vi "Main.vi"(11 "Module Admin":refnum<class "Delacor_lib_QMH_Module Admin.lvclass">) -> ()   [LabVIEW 2019, in "Settings Editor.lvlib"]
doc: "This template is based off of the Queued Message Handler design pattern and the Queued Message Handler project template that ships with LabVIEW.\n\nThe main difference is that the queue is private to this module and communication between modules is performed via Broadcast and Request events.\n\nRequest events are wrapped in public API methods and are handled in the Event Handling Loop (EHL) of this VI. Any module can register for Broadcast events sent by this module. The EHL generates messages based on user interface actions.\n\nThe Message Handling Loop (MHL) processes messages generated by the EHL, or by other messages. The messages are string values, so new messages can be added easily to the Message Cases case structure in the MHL. Each message cluster can also provide an optional value for Message Data, which is a variant that can be converted to whatever message-specific data is required.\n_____\nBased on Delacor QMH Project Template 4.0.0.47.\n_____\nBased on DQMH Project Template 6.1.0.94."
uses:
  Settings Editor.lvlib
  <vilib>/Delacor/Delacor QMH/Libraries/Module Admin_class/Delacor_lib_QMH_Module Admin.lvclass
  Module Data--cluster.ctl
  Settings--cluster.ctl
  Stop Argument--cluster.ctl
  <vilib>/Delacor/Delacor QMH/Libraries/Message Queue_class/Delacor_lib_QMH_Message Queue.lvclass/Delacor_lib_QMH_Message Queue.ctl
  <vilib>/Delacor/Delacor QMH/Libraries/Module Admin_class/Delacor_lib_QMH_Module Admin.lvclass/Delacor_lib_QMH_Module Admin.ctl
  <vilib>/Utility/miscctls.llb/LVPointTypeDef.ctl
  <vilib>/Delacor/Delacor QMH/Libraries/Message Queue_class/Delacor_lib_QMH_Enqueue Message (Single).vi
  <vilib>/Delacor/Delacor QMH/Libraries/Module Admin_class/Delacor_lib_QMH_Get External Launch.vi
  <vilib>/Utility/error.llb/Error Cluster From Error Code.vi
  <vilib>/ErrorRing/Error Ring.xnode
  <vilib>/Delacor/Delacor QMH/Libraries/Message Queue_class/Delacor_lib_QMH_Message Queue.lvclass
panel:
  in  "Dir?":bool=TRUE
  in  "TDMS Directory":path
  in  "Cancel":bool
  in  "OK":bool
  in  "TDMS filepath":path
  out "error out":errorcluster
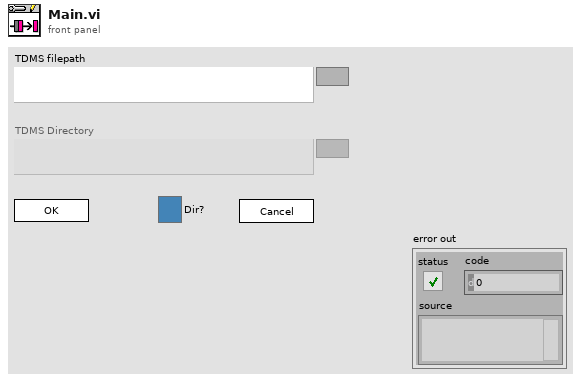
[diagram p1: front panel]
types:
  T1 = typedef "Settings Editor.lvlib/Request Events--cluster.ctl" = cluster{"Stop Module":refnum<user-event>, "Show Panel":refnum<user-event>, "Hide Panel":refnum<user-event>, "Get Module Execution Status":refnum<user-event>, "Show Diagram":refnum<user-event>}
  T2 = typedef "Settings Editor.lvlib/Module Data--cluster.ctl" = cluster{"Settings":T3}
  T3 = typedef "Settings Editor.lvlib/Settings--cluster.ctl" = cluster{"TDMS Filepath":path, "TDMS Directory":path}
  T4 = enum32{"invalid lock state", "Not Locked", "Locked (No Password)", "Password-protected"}
  T5 = typedef "Settings Editor.lvlib/Stop Argument--cluster.ctl" = cluster{"Origin":string, "Exit via Stop Module Req?":bool, "Wait for Module to stop?":bool}
  T6 = typedef "LVPointTypeDef.ctl" = cluster{"Horizontal":i16, "Vertical":i16}
  T7 = enum32{"Invalid", "Standard", "Closed", "Hidden", "Minimized", "Maximized"}
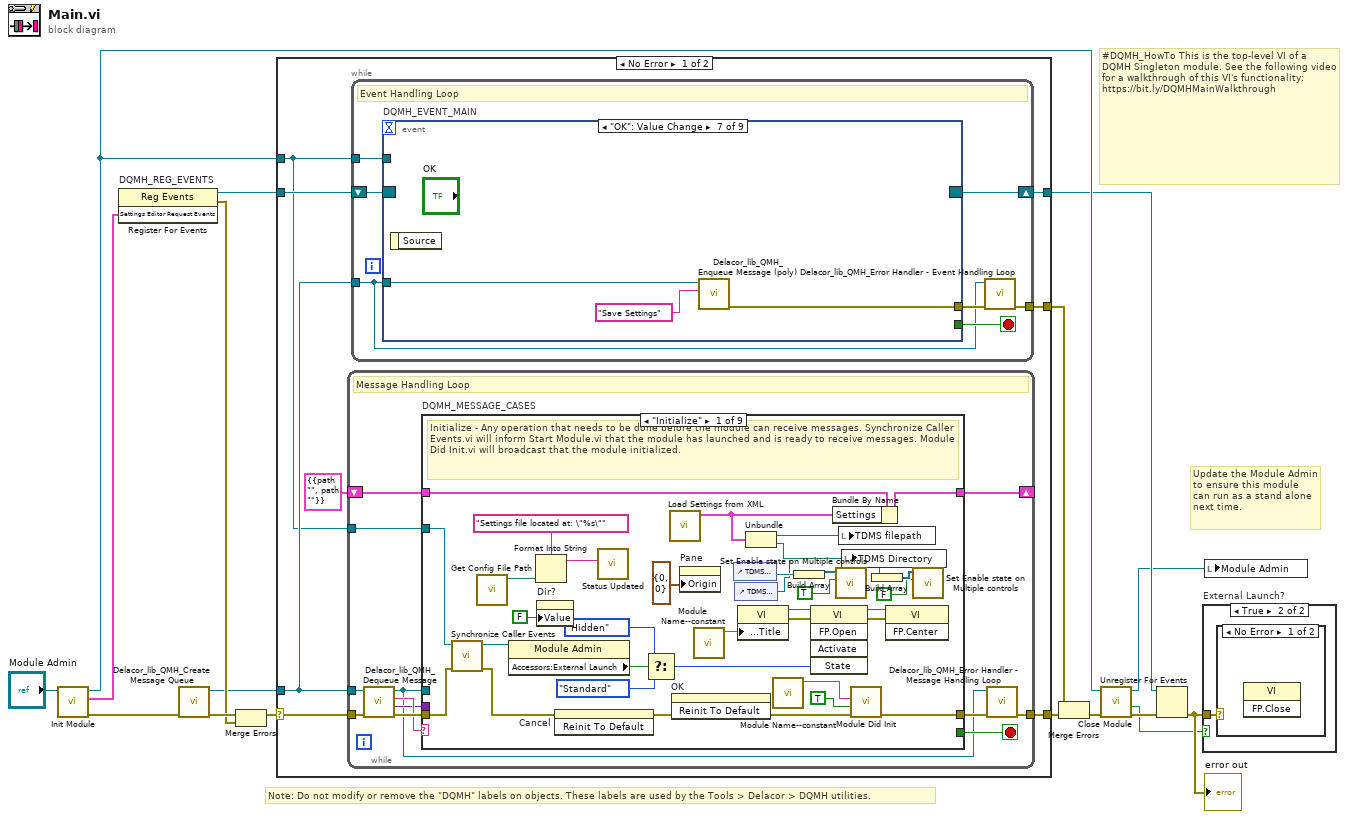
[diagram p0: block diagram]
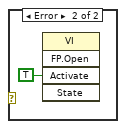
[diagram p3: hidden frame]
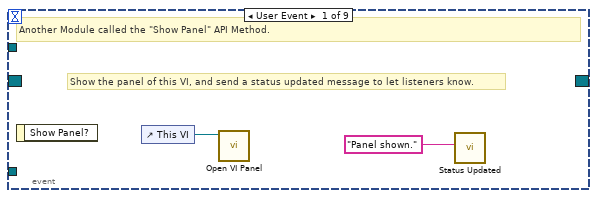
[diagram p4: hidden frame]
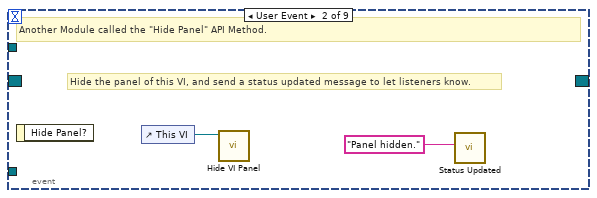
[diagram p5: hidden frame]
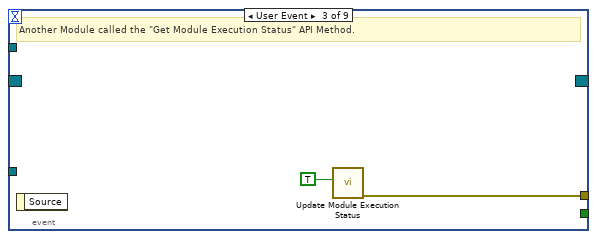
[diagram p6: hidden frame]
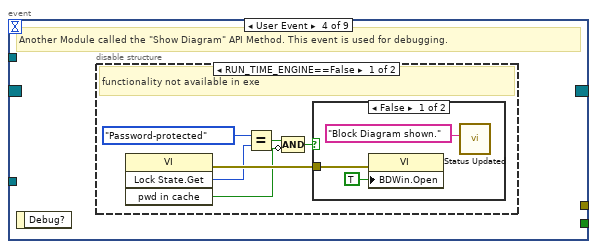
[diagram p7: hidden frame]
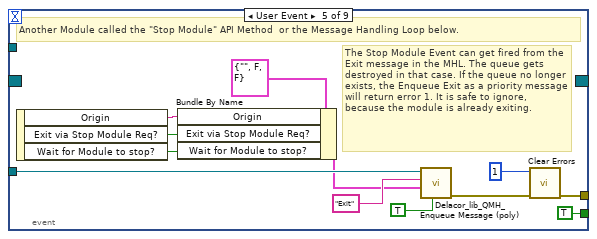
[diagram p10: hidden frame]
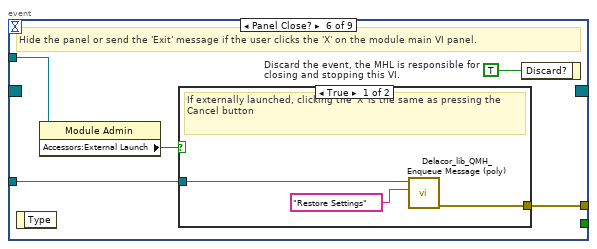
[diagram p11: hidden frame]
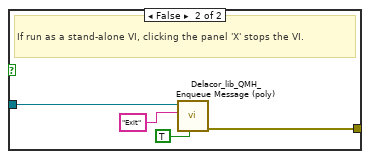
[diagram p12: hidden frame]
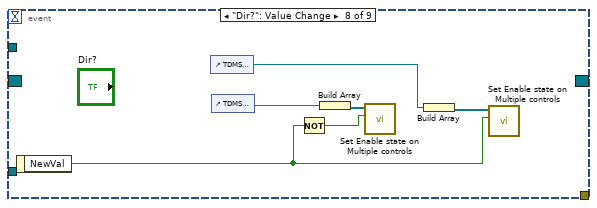
[diagram p13: hidden frame]
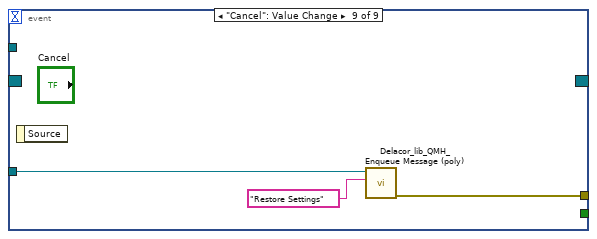
[diagram p14: hidden frame]
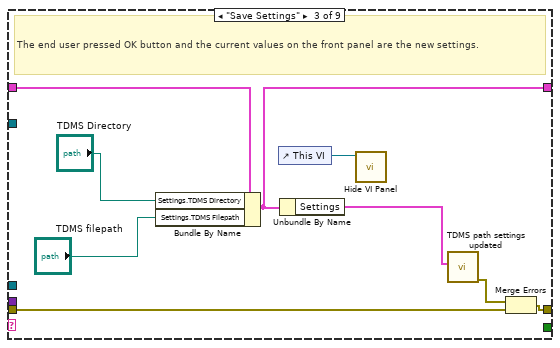
[diagram p16: hidden frame]
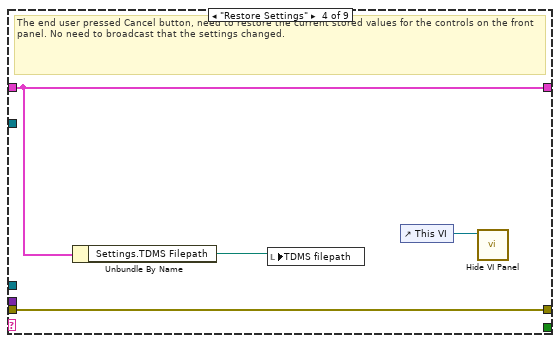
[diagram p17: hidden frame]
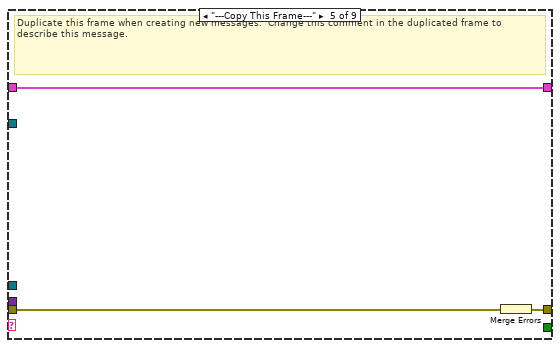
[diagram p18: hidden frame]
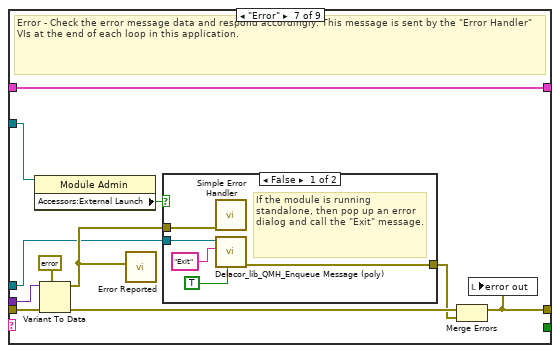
[diagram p20: hidden frame]
diagram:
  # "#DQMH_HowTo This is the top-level VI of a DQMH Singleton module. See the following video for a walkthrough of this VI's functionality: https://bit.ly/DQMHMainWalkthrough"
  # "Note: Do not modify or remove the \"DQMH\" labels on objects. These labels are used by the Tools > Delacor > DQMH utilities."
  # "Update the Module Admin to ensure this module can run as a stand alone next time."
  n1 = call "Init Module.vi"("Singleton Module Admin in"="Module Admin") -> ("error out"=w16:errorcluster, "Settings Editor Request Events"=w5:T1, "Singleton Module Admin out"=w8:refnum<class "Delacor_lib_QMH_Module Admin.lvclass">)  [unwired: 8 in]
  n2 = register-events "DQMH_REG_EVENTS"(w5) -> (reference out=w6:refnum<event-registration>, error out=w9:errorcluster)  [unwired: 2 in]
  n3 = call <vilib>:"Delacor_lib_QMH_Create Message Queue.vi"("error in"=w16) -> ("error out"=w11:errorcluster, "Message Queue"=w4:refnum<class "Delacor_lib_QMH_Message Queue.lvclass">)  [unwired: 9 in]
  n4 = Merge Errors(w11, w9) -> (w10:errorcluster)
  n5 = case shown="No Error" w10 {
    selector: w10 -> [w23 w194]
    tunnel: [w25 w193] -> w17
    tunnel: [w22 w200] -> w7
    tunnel: w6 -> [w20 w200]
    tunnel: w4 -> [w19 w195]
    tunnel: [w24 _] -> w14
    tunnel: w8 -> [w18 w196]
    frame No Error {
      n6 = while {
        tunnel: w19 -> [w86]
        shift-right: [w90] -> _
        shift-left: T2 {"Settings"={"TDMS Filepath"=path "", "TDMS Directory"=path ""}} ("Data Cluster") -> [w91]
        tunnel: w23 -> [w94]
        tunnel: [w92] -> w25
        tunnel: w18 -> [w84]
        stop <- w89 stop-if-true
        # "Message Handling Loop"
        n7 = call-dynamic "Delacor_lib_QMH_Dequeue Message.vi"("error in"=w94, "Message Queue in"=w86) -> ("error out"=w93:errorcluster, "Message Data"=w87:variant, "Message"=w88:string, "Message Queue out"=w85:refnum<class "Delacor_lib_QMH_Message Queue.lvclass">)  [unwired: 6 in]
        n8 = case "DQMH_MESSAGE_CASES" shown="\"Initialize\"" w88 {
          selector: w88 -> [_ _ _ _ _ _ _ _ w180]
          tunnel: w85 -> [_ _ _ _ _ _ w150 w172 _]
          tunnel: w93 -> [w126 w129 w133 w142 w145 w147 w157 w178 w182]
          tunnel: [w124 w129 w134 w142 w144 w147 w153 w175 w183] -> w95
          tunnel: w91 -> [w115 w128 w138 w141 w143 w146 w152 w171 w181]
          tunnel: [w114 w128 w136 w141 w143 w146 w152 w171 w181] -> w90
          tunnel: [_ _ _ _ _ _ _ w170 _] -> w89
          tunnel: w87 -> [_ _ _ _ _ _ w151 w169 _]
          tunnel: w84 -> [w116 _ _ _ _ _ w149 w164 _]
          frame "Initialize" {
            # "Initialize - Any operation that needs to be done before the module can receive messages. Synchronize Caller Events.vi will inform Start Module.vi that the module has launched and is ready to receive messages. Module Did Init.vi will broadcast that the module initialized."
            n9 = call "Synchronize Caller Events.vi"("error in (no error)"=w126, "Singleton Module Admin in"=w116) -> ("error out"=w125:errorcluster, "Singleton Module Admin out"=w111:refnum<class "Delacor_lib_QMH_Module Admin.lvclass">)  [unwired: 8 in]
            n10 = call "Get Config File Path.vi"() -> ("XML File Path"=w108:path)  [unwired: 10 in, 1 out]
            n11 = property class="Module Admin"(reference=w111) -> ("Accessors:External Launch"=w120:bool)  [unwired: 1 in, 2 out]
            n12 = Format Into String(format string="Settings file located at: \"%s\"", w108) -> (resulting string=w107:string)  [unwired: 2 in, 1 out]
            n13 = property on="Dir?" class="Bool (strict)"("Value"=FALSE ("Dir?")) -> ()  [unwired: 2 in, 2 out]
            n14 = invoke on="Cancel" class="Bool" method="Reinit To Default"() -> ()  [unwired: 3 in, 3 out]
            n15 = call "Status Updated.vi"("Status"=w107) -> ()  [unwired: 10 in, 1 out]
            n16 = Select(t=T7."Hidden" ("State"), s=w120, f=T7."Standard" ("State")) -> (s? t:f=w117:T7)
            n17 = call "Load Settings from XML.vi"() -> ("Settings out"=w105:T3)  [unwired: 10 in, 1 out]
            n18 = invoke on="OK" class="Bool" method="Reinit To Default"() -> ()  [unwired: 3 in, 3 out]
            n19 = property on="Pane" class="Pane"("Origin"=T6 {"Horizontal"=0, "Vertical"=0}) -> ()  [unwired: 2 in, 2 out]
            n20 = call "Module Name--constant.vi"() -> ("Module Name"=w123:string)  [unwired: 11 in]
            n21 = control-ref of="TDMS filepath"() -> (w102:refnum<vi>)
            n22 = control-ref of="TDMS Directory"() -> (w101:refnum<vi>)
            n23 = property class="VI"("Front Panel.Title"=w123) -> (reference out=w122:refnum<vi>, error out=w109:errorcluster)  [unwired: 2 in]
            n24 = Unbundle(w105) -> ("TDMS Filepath"=w104:path, "TDMS Directory"=w103:path)
            n25 = call "Module Name--constant.vi"() -> ("Module Name"=w112:string)  [unwired: 11 in]
            n26 = Build Array(w102) -> (w100:refnum<vi>[])
            n27 = invoke class="VI" method="FP.Open"(reference=w122, error in=w109, "State"=w117) -> (reference out=w121:refnum<vi>, error out=w127:errorcluster)  [unwired: 2 in, 3 out]
            n28 = Bundle By Name(cluster=w115, "Settings"=w105) -> (w114:T2)
            n29 = call "Set Enable state on Multiple controls.vi"("Enable?"=TRUE, "Controls"=w100) -> ()  [unwired: 10 in]
            n30 = local write "TDMS filepath"(w104) -> ()
            n31 = local write "TDMS Directory"(w103) -> ()
            n32 = call "Module Did Init.vi"("error in (no error)"=w125, "Initialized?"=TRUE, "Origin"=w112) -> ("error out"=w124:errorcluster)  [unwired: 8 in]
            n33 = Build Array(w101) -> (w99:refnum<vi>[])
            n34 = invoke class="VI" method="FP.Center"(reference=w121, error in=w127) -> ()  [unwired: 1 in, 3 out]
            n35 = call "Set Enable state on Multiple controls.vi"("Enable?"=FALSE, "Controls"=w99) -> ()  [unwired: 10 in]
          }
          frame "---Module Specific---" {
            # "Separator -- The following cases handle messages specific to this Module."
          }
          frame "Save Settings" {
            # "The end user pressed OK button and the current values on the front panel are the new settings."
            n36 = Bundle By Name(cluster=w138, "Settings.TDMS Directory"="TDMS Directory", "Settings.TDMS Filepath"="TDMS filepath") -> (w136:T2)
            n37 = control-ref of="This VI"() -> (w137:refnum<vi>)
            n38 = Unbundle By Name(w136) -> ("Settings"=w130:T3)
            n39 = call "Hide VI Panel.vi"("VI"=w137) -> ()  [unwired: 10 in, 1 out]
            n40 = call "TDMS path settings updated.vi"("Settings"=w130) -> ("error out"=w131:errorcluster)  [unwired: 10 in]
            n41 = Merge Errors(w131, w133) -> (w134:errorcluster)
          }
          frame "Restore Settings" {
            # "The end user pressed Cancel button, need to restore the current stored values for the controls on the front panel. No need to broadcast that the settings changed."
            n42 = Unbundle By Name(w141) -> ("Settings.TDMS Filepath"=w140:path)
            n43 = local write "TDMS filepath"(w140) -> ()
            n44 = control-ref of="This VI"() -> (w139:refnum<vi>)
            n45 = call "Hide VI Panel.vi"("VI"=w139) -> ()  [unwired: 10 in, 1 out]
          }
          frame "---Copy This Frame---" {
            # "Duplicate this frame when creating new messages.  Change this comment in the duplicated frame to describe this message."
            n46 = Merge Errors(w145) -> (w144:errorcluster)
          }
          frame "---Exit and Error Handling---" {
            # "Separator - The following cases handle errors and exit messages."
          }
          frame "Error" {
            # "Error - Check the error message data and respond accordingly. This message is sent by the \"Error Handler\" VIs at the end of each loop in this application."
            n47 = property class="Module Admin"(reference=w149) -> ("Accessors:External Launch"=w148:bool)  [unwired: 1 in, 2 out]
            n48 = Variant To Data(error in=w157, type=errorcluster {"status"=FALSE, "code"=0, "source"=""} ("error constant"), Variant=w151) -> (data=w158:errorcluster, error out=w155:errorcluster)
            n49 = call "Error Reported.vi"("Error"=w158) -> ()  [unwired: 10 in, 1 out]
            n50 = case shown="False" w148 {
              tunnel: [w163 _] -> w154
              tunnel: w150 -> [w161 _]
              tunnel: w158 -> [w162 _]
              frame False {
                # "If the module is running standalone, then pop up an error dialog and call the \"Exit\" message."
                n51 = call <vilib>:"Simple Error Handler.vi"("error in (no error)"=w162) -> ()  [unwired: 4 in, 5 out]
                n52 = call-poly <vilib>:"Delacor_lib_QMH_Enqueue Message (poly).vi"("Priority Message? (F)"=TRUE, "Message"="Exit", "Message Queue in"=w161) -> ("error out"=w163:errorcluster)  [unwired: 7 in, 1 out]
              }
              frame True {
                # "If the module was launched externally, calling the Error Reported broadcast VI is the only action performed by the \"Error\" message. The module's caller can then process the error appropriately."
              }
            }
            n53 = Merge Errors(w155, w154) -> (w153:errorcluster)
            n54 = local write "error out"(w153) -> ()
          }
          frame "Exit" {
            w168 = 91  # 91: not all Exit messages will have an argument
            w170 = TRUE  # Stop the VI
            # "Release the message queue reference"
            # "Exit - Exit the application."
            n55 = Variant To Data(error in=w178, type=T5 {"Origin"="", "Exit via Stop Module Req?"=FALSE, "Wait for Module to stop?"=FALSE} ("Stop Argument"), Variant=w169) -> (data=w166:T5, error out=w174:errorcluster)
            n56 = call <vilib>:"Clear Errors.vi"("error in (no error)"=w174, "specific error code to clear (0: all)"=w168) -> ("error out"=w177:errorcluster)  [unwired: 4 in, 1 out]
            n57 = control-ref of="This VI"() -> (w165:refnum<vi>)
            n58 = call-dynamic "Delacor_lib_QMH_Release Message Queue.vi"("error in"=w177, "Message Queue"=w172) -> ("error out"=w176:errorcluster)  [unwired: 9 in]
            n59 = call "Handle Exit.vi"("Stop Argument"=w166, "Admin in"=w164, "VI reference"=w165) -> ("error out"=w173:errorcluster)  [unwired: 7 in, 1 out]
            n60 = Merge Errors(w176, w173) -> (w175:errorcluster)
          }
          frame Default {
            # "'Default' case only runs if there is a message that isn't defined in any of the other cases.  Output a programming error."
            n61 = call "Module Name--constant.vi"() -> ("Module Name"=w179:string)  [unwired: 11 in]
            n62 = xnode "Error Ring"("parameter 0"=w180, "parameter 1"=w179) -> ("error out"=w184:errorcluster)
            n63 = Merge Errors(w182, w184) -> (w183:errorcluster)
          }
        }
        n64 = call-dynamic "Delacor_lib_QMH_Error Handler - Message Handling Loop.vi"("error in"=w95, "Message Queue in"=w85) -> ("dup error in"=w92:errorcluster)  [unwired: 8 in, 1 out]
      }
      n65 = while {
        tunnel: w19 -> [w26]
        shift-right: [w29] -> w22
        shift-left: w20 -> [w30]
        tunnel: [w31] -> w24
        tunnel: w18 -> [w27]
        stop <- w28 stop-if-true
        # "Event Handling Loop"
        n66 = event "DQMH_EVENT_MAIN" shown="[6] \"OK\": Value Change" {
          selector: w30 -> [_ _ _ _ _ _ _ _ _]
          dyn-events: [_ _ _ _ _ _ _ _ _] -> w29
          timeout: _ -> [_ _ _ _ _ _ _ _ _]
          tunnel: [_ _ _ _ TRUE ("Discard?") _ _ _ _] -> w28
          tunnel: w26 -> [_ _ _ _ w55 w62 w72 _ w82]
          tunnel: [_ _ w38 _ w58 w64 w73 _ w81] -> w32
          tunnel: w27 -> [_ _ _ _ _ w61 _ _ _]
          event User Event {
            # "Show the panel of this VI, and send a status updated message to let listeners know."
            # "Another Module called the \"Show Panel\" API Method."
            n67 = event-data() -> ()  [unwired: 1 in, 1 out]
            n68 = control-ref of="This VI"() -> (w34:refnum<vi>)
            n69 = call "Open VI Panel.vi"("VI"=w34) -> ()  [unwired: 10 in, 1 out]
            n70 = call "Status Updated.vi"("Status"="Panel shown." ("format string")) -> ()  [unwired: 10 in, 1 out]
          }
          event User Event {
            # "Hide the panel of this VI, and send a status updated message to let listeners know."
            # "Another Module called the \"Hide Panel\" API Method."
            n71 = event-data() -> ()  [unwired: 1 in, 1 out]
            n72 = control-ref of="This VI"() -> (w36:refnum<vi>)
            n73 = call "Hide VI Panel.vi"("VI"=w36) -> ()  [unwired: 10 in, 1 out]
            n74 = call "Status Updated.vi"("Status"="Panel hidden." ("format string")) -> ()  [unwired: 10 in, 1 out]
          }
          event User Event {
            # "Another Module called the \"Get Module Execution Status\" API Method."
            n75 = event-data() -> ()  [unwired: 1 in, 1 out]
            n76 = call "Update Module Execution Status.vi"("Running?"=TRUE) -> ("error out"=w38:errorcluster)  [unwired: 10 in]
          }
          event User Event {
            # "Another Module called the \"Show Diagram\" API Method. This event is used for debugging."
            n77 = event-data() -> ()  [unwired: 1 in, 1 out]
            n78 = disable-structure shown="RUN_TIME_ENGINE==False" {
              frame condition #0 (active) {
                # "functionality not available in exe"
                n79 = invoke class="VI" method="Lock State.Get"() -> (error out=w44:errorcluster, "Get Lock State"=w43:T4, "pwd in cache"=w40:bool)  [unwired: 4 in, 1 out]
                n80 = Equal?(x=T4."Password-protected", y=w43) -> (x = y?=w41:bool)
                n81 = Compound Arithmetic op=AND(w41, invert w40) -> (w39:bool)
                n82 = case shown="False" w39 {
                  tunnel: w44 -> [w47 _]
                  frame False {
                    n83 = property class="VI"(error in=w47, "BDWin.Open"=TRUE ("Block Diagram Window:Open")) -> ()  [unwired: 1 in, 2 out]
                    n84 = call "Status Updated.vi"("Status"="Block Diagram shown." ("format string")) -> ()  [unwired: 10 in, 1 out]
                  }
                  frame True {
                    # "Password-protected VI, and the password is not in the cache. Do not show the diagram."
                  }
                }
              }
              frame condition #1 {
              }
            }
          }
          event User Event {
            # "The Stop Module Event can get fired from the Exit message in the MHL. The queue gets destroyed in that case. If the queue no longer exists, the Enqueue Exit as a priority message will return error 1. It is safe to ignore, because the module is already exiting."
            # "Another Module called the \"Stop Module\" API Method  or the Message Handling Loop below."
            n85 = event-data() -> ("Origin"=w48:string, "Exit via Stop Module Req?"=w51:bool, "Wait for Module to stop?"=w50:bool)  [unwired: 1 in]
            n86 = Bundle By Name(cluster=T5 {"Origin"="", "Exit via Stop Module Req?"=FALSE, "Wait for Module to stop?"=FALSE} ("Stop Argument"), "Origin"=w48, "Exit via Stop Module Req?"=w51, "Wait for Module to stop?"=w50) -> (w49:T5)
            n87 = call-poly <vilib>:"Delacor_lib_QMH_Enqueue Message (poly).vi"("Priority Message? (F)"=TRUE, "Message Data"=w49, "Message"="Exit", "Message Queue in"=w55) -> ("error out"=w59:errorcluster)  [unwired: 6 in, 1 out]
            n88 = call <vilib>:"Clear Errors.vi"("error in (no error)"=w59, "specific error code to clear (0: all)"=1) -> ("error out"=w58:errorcluster)  [unwired: 4 in, 1 out]
          }
          event Panel Close? {
            w63 = TRUE  # Discard the event, the MHL is responsible for closing and stopping this VI.
            # "Hide the panel or send the 'Exit' message if the user clicks the 'X' on the module main VI panel."
            n89 = event-data() -> ()  [unwired: 1 in, 1 out]
            n90 = property class="Module Admin"(reference=w61) -> ("Accessors:External Launch"=w60:bool)  [unwired: 1 in, 2 out]
            n91 = case shown="True" w60 {
              tunnel: w62 -> [w66 w70]
              tunnel: [w65 w71] -> w64
              frame True {
                # "If externally launched, clicking the 'X' is the same as pressing the Cancel button"
                n92 = call-poly <vilib>:"Delacor_lib_QMH_Enqueue Message (poly).vi"("Message"="Restore Settings", "Message Queue in"=w66) -> ("error out"=w65:errorcluster)  [unwired: 8 in, 1 out]
              }
              frame False {
                # "If run as a stand-alone VI, clicking the panel 'X' stops the VI."
                n93 = call-poly <vilib>:"Delacor_lib_QMH_Enqueue Message (poly).vi"("Priority Message? (F)"=TRUE, "Message"="Exit", "Message Queue in"=w70) -> ("error out"=w71:errorcluster)  [unwired: 7 in, 1 out]
              }
            }
            n94 = event-data("Discard?"=w63) -> ()  [unwired: 1 in, 1 out]
          }
          event "OK": Value Change {
            n95 = event-data() -> ()  [unwired: 1 in, 1 out]
            n96 = call-poly <vilib>:"Delacor_lib_QMH_Enqueue Message (poly).vi"("Message"="Save Settings", "Message Queue in"=w72) -> ("error out"=w73:errorcluster)  [unwired: 8 in, 1 out]
          }
          event "Dir?": Value Change {
            n97 = event-data() -> ("NewVal"=w75:bool)  [unwired: 1 in]
            n98 = control-ref of="TDMS Directory"() -> (w80:refnum<vi>)
            n99 = control-ref of="TDMS filepath"() -> (w78:refnum<vi>)
            n100 = Not(x=w75) -> (.not. x?=w76:bool)
            n101 = Build Array(w78) -> (w77:refnum<vi>[])
            n102 = call "Set Enable state on Multiple controls.vi"("Enable?"=w76, "Controls"=w77) -> ()  [unwired: 10 in]
            n103 = Build Array(w80) -> (w79:refnum<vi>[])
            n104 = call "Set Enable state on Multiple controls.vi"("Enable?"=w75, "Controls"=w79) -> ()  [unwired: 10 in]
          }
          event "Cancel": Value Change {
            n105 = event-data() -> ()  [unwired: 1 in, 1 out]
            n106 = call-poly <vilib>:"Delacor_lib_QMH_Enqueue Message (poly).vi"("Message"="Restore Settings", "Message Queue in"=w82) -> ("error out"=w81:errorcluster)  [unwired: 8 in, 1 out]
          }
        }
        n107 = call-dynamic "Delacor_lib_QMH_Error Handler - Event Handling Loop.vi"("error in"=w32, "Message Queue in"=w26) -> ("dup error in"=w31:errorcluster)  [unwired: 8 in, 1 out]
      }
    }
    frame Error {
      # "Synchronize Caller Events.vi will inform Start Module.vi that the module has launched and will let the code calling Start Module.vi register for broadcasts and would permit the caller receive the broadcast that an error occurred at launch time."
      n108 = call "Synchronize Caller Events.vi"("Singleton Module Admin in"=w196) -> ("error out"=w201:errorcluster)  [unwired: 9 in, 1 out]
      n109 = call-dynamic "Delacor_lib_QMH_Release Message Queue.vi"("error in"=w194, "Message Queue"=w195) -> ("error out"=w193:errorcluster)  [unwired: 9 in]
      n110 = call "Module Name--constant.vi"() -> ("Module Name"=w199:string)  [unwired: 11 in]
      n111 = Format Into String(format string="An error occurred during initialization. %s is no longer running.", w199) -> (resulting string=w197:string)  [unwired: 2 in, 1 out]
      n112 = Merge Errors(w193, w201) -> (w202:errorcluster)
      n113 = call "Error Reported.vi"("Additional Information"=w197, "Error"=w202) -> ()  [unwired: 9 in, 1 out]
    }
  }
  n114 = Merge Errors(w14, w17) -> (w13:errorcluster)
  n115 = call "Close Module.vi"("error in (no error)"=w13, "Module Admin in"=w8) -> ("error out"=w15:errorcluster, "External Launch"=w1:bool, "Module Admin out"=w2:refnum<class "Delacor_lib_QMH_Module Admin.lvclass">)  [unwired: 7 in]
  n116 = Unregister For Events(event registration refnum=w7, error in=w15) -> (error out=w12:errorcluster)
  "error out" <- w12
  n117 = case "External Launch?" shown="True" w1 {
    tunnel: w12 -> [_ w203]
    frame False {
    }
    frame True {
      n118 = case shown="No Error" w203 {
        frame No Error {
          n119 = invoke class="VI" method="FP.Close"() -> ()  [unwired: 3 in, 3 out]
        }
        frame Error {
          n120 = invoke class="VI" method="FP.Open"("Activate"=TRUE ("Activate?")) -> ()  [unwired: 4 in, 5 out]
        }
      }
    }
  }
  n121 = local write "Module Admin"(w2) -> ()
